vi "REP-REQ TCP.vi"(7 "TcpRouter-Client in":refnum<class "TcpRouter-Client.lvclass">, 8 "error in (no error)":errorcluster) -> (0 "error out":errorcluster, 2 "REQ-REP":refnum<data-value>, 3 "connection ID":refnum<k5>)   [LabVIEW 2020, in "CSM-TCP-Router.lvlib" / "TcpRouter-Client.lvclass"]
uses:
  TcpRouter-Client.lvclass
  Def-TCP-Router REQ-REP.ctl
  TcpRouter-Client.lvclass/TcpRouter-Client.ctl
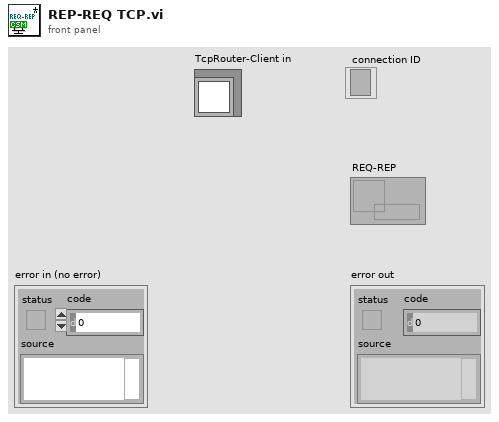
[diagram p1: front panel]
types:
  T1 = cluster{"IP Address":string, "Port":u16, "ConnectTMO":i32}
  T2 = typedef "CSM-TCP-Router.lvlib/TcpRouter-Client.lvclass/Def-TCP-Router REQ-REP.ctl" = cluster{"REQ-REP":refnum<k5>}
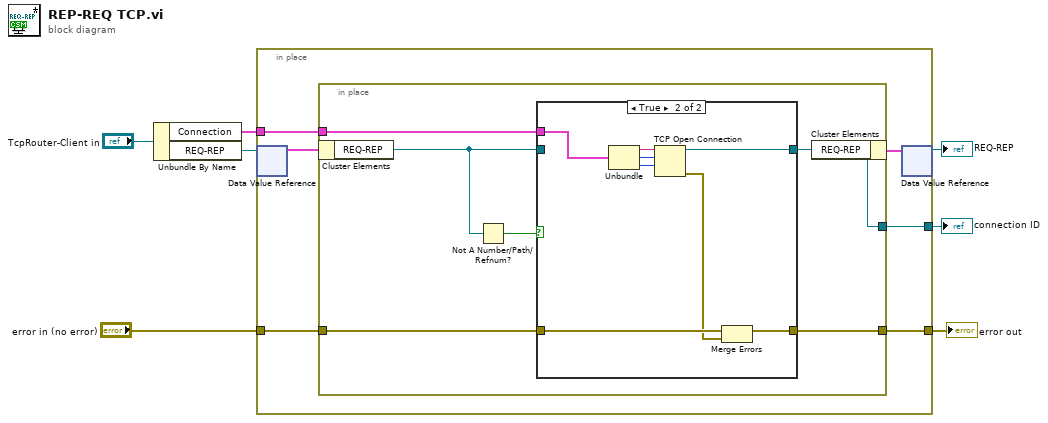
[diagram p0: block diagram]
diagram:
  n1 = Unbundle By Name("TcpRouter-Client in") -> ("Connection"=w3:T1, "REQ-REP"=w4:refnum<data-value>)
  n2 = in-place {
    in-place-border: w3 -> [w11]
    in-place-border: [w10] -> w6
    in-place-border: "error in (no error)" -> [w9]
    in-place-border: [w8] -> w2
    n3 = in-place-dvr #1(w4) -> (w13:T2)  [unwired: 1 out]
    n4 = in-place {
      in-place-border: w11 -> [w19]
      in-place-border: [w17] -> w10
      in-place-border: w9 -> [w18]
      in-place-border: [w14] -> w8
      n5 = in-place-cluster #2(w13) -> ("REQ-REP"=w15:refnum<k5>)
      n6 = Not A Number/Path/Refnum?(number/path/refnum=w15) -> (NaN/Path/Refnum?=w16:bool)
      n7 = case shown="True" w16 {
        tunnel: w19 -> [_ w27]
        tunnel: w18 -> [w20 w26]
        tunnel: [w20 w25] -> w17
        tunnel: [w21 w23] -> w14
        tunnel: w15 -> [w21 _]
        frame False {
        }
        frame True {
          n8 = Unbundle(w27) -> ("IP Address"=w29:string, "Port"=w28:u16, "ConnectTMO"=w22:i32)
          n9 = TCP Open Connection(address=w29, remote port or service name=w28, timeout ms (60000)=w22) -> (connection ID=w23:refnum<k5>, error out=w24:errorcluster)  [unwired: 2 in]
          n10 = Merge Errors(w26, w24) -> (w25:errorcluster)
        }
      }
      n11 = in-place-cluster #2("REQ-REP"=w14) -> (w12:T2)
    }
    n12 = in-place-dvr #1(w12) -> (→"REQ-REP":refnum<data-value>)  [unwired: 1 out]
  }
  "error out" <- w6
  "connection ID" <- w2
